vi "test.vi"() -> ()   [LabVIEW 2018]
uses:
  <vilib>/Analysis/coordinate.llb/2D Cartesian Coordinate Rotation (Scalar).vi
  <vilib>/Analysis/NI_AALPro.lvlib
panel:
  out "POS N":dbl[](array[numeric])
  in  "POS":dbl[](array[numeric])
  out "x out 2":dbl
  in  "theta 2":dbl
  in  "X":dbl
  in  "X1":dbl
  in  "Y1":dbl
  in  "X2":dbl
  in  "Y2":dbl
  out "r":dbl
  out "theta":dbl
  in  "RAD":dbl
  out "x out":dbl
  out "y out":dbl
  out "Head":dbl
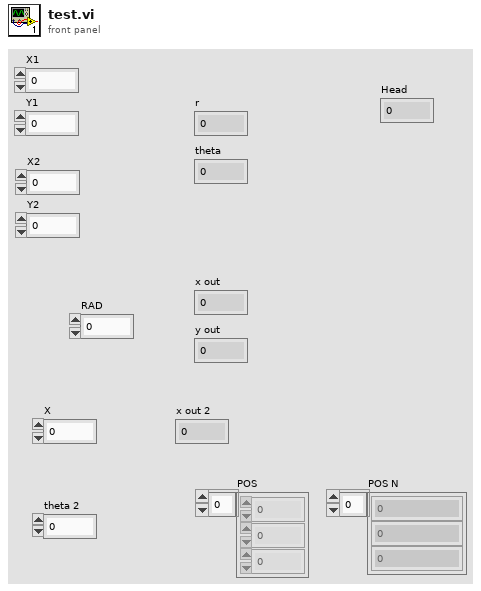
[diagram p1: front panel]
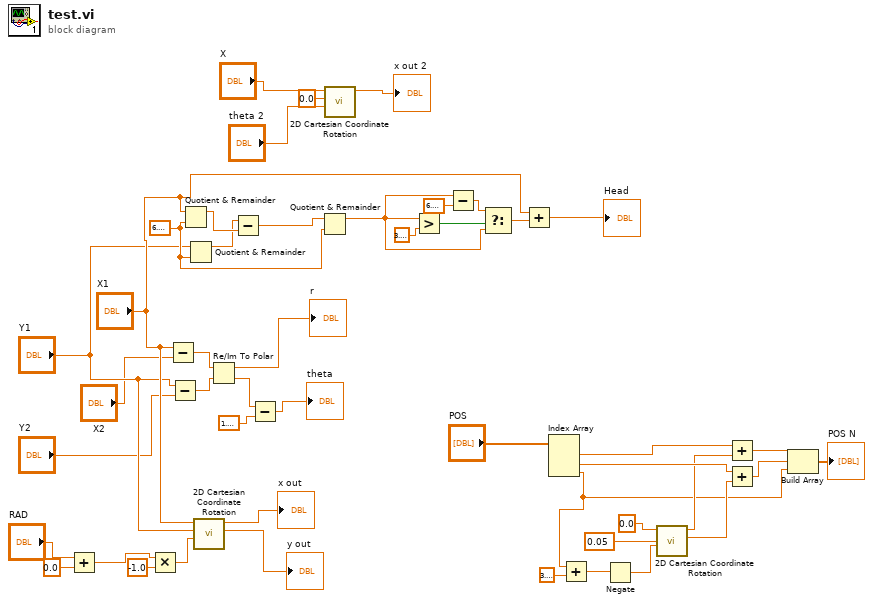
[diagram p0: block diagram]
diagram:
  w38 = 6.283185307179586
  n1 = Add(x="RAD", y=0.0) -> (x+y=w32:dbl)
  n2 = Multiply(x=w32, y=-1.0) -> (x*y=w29:dbl)
  n3 = Subtract(x="X1", y="X2") -> (x-y=w20:dbl)
  n4 = Subtract(x="Y1", y="Y2") -> (x-y=w19:dbl)
  n5 = Quotient & Remainder(x="X1", y=w38) -> (x-y*floor(x/y)=w35:dbl)  [unwired: 1 out]
  n6 = Quotient & Remainder(x="Y1", y=w38) -> (x-y*floor(x/y)=w34:dbl)  [unwired: 1 out]
  n7 = call-poly <vilib>:"2D Cartesian Coordinate Rotation.vi"("theta"=w29, "y"="Y1", "x"="X1") -> ("y out"=→"y out":dbl, "x out"=→"x out":dbl)  [unwired: 6 in, 1 out]
  n8 = Re/Im To Polar(2:w19, 3:w20) -> (0:w24:dbl, 1:→"r":dbl)
  n9 = Subtract(x=w34, y=w35) -> (x-y=w37:dbl)
  n10 = Subtract(x=w24, y=1.5707963267948966) -> (x-y=→"theta":dbl)
  n11 = Quotient & Remainder(x=w37, y=w38) -> (x-y*floor(x/y)=w43:dbl)  [unwired: 1 out]
  n12 = call-poly <vilib>:"2D Cartesian Coordinate Rotation.vi"("theta"="theta 2", "y"=0.0, "x"="X") -> ("x out"=→"x out 2":dbl)  [unwired: 6 in, 2 out]
  n13 = Greater?(x=w43, y=3.141592653589793) -> (0:w40:bool)
  n14 = Subtract(x=w43, y=6.283185307179586) -> (x-y=w42:dbl)
  n15 = Select(t=w42, s=w40, f=w43) -> (s? t:f=w44:dbl)
  n16 = Add(x="X1", y=w44) -> (x+y=→"Head":dbl)
  n17 = Index Array(array="POS") -> (element #1=w11:dbl, element #2=w10:dbl, element #3=w4:dbl)  [unwired: 3 in]
  n18 = Add(x=w4, y=3.141592653589793) -> (x+y=w2:dbl)
  n19 = Negate(x=w2) -> (-x=w1:dbl)
  n20 = call-poly <vilib>:"2D Cartesian Coordinate Rotation.vi"("theta"=w1, "y"=0.05, "x"=0.0) -> ("y out"=w8:dbl, "x out"=w9:dbl)  [unwired: 6 in, 1 out]
  n21 = Add(x=w11, y=w9) -> (x+y=w6:dbl)
  n22 = Add(x=w10, y=w8) -> (x+y=w5:dbl)
  n23 = Build Array(w6, w5, w4) -> (→"POS N":dbl[])
